vi "Testing.vi"() -> ()   [LabVIEW 2021]
uses:
  Motion_Panel_State_Machine/Motion_Panel_State_Machine.lvclass
  C:/Program Files (x86)/Hyper State Machine Framework/Hyper_Panel_State_Machine_Adaptive.lvlibp/Hyper Panel State Machine Object_Adaptive_2021/Hyper_Panel_State_Machine/Hyper_Panel_State_Machine_Adaptive.lvclass
  DIO_Panel_State_Machine/DIO_Panel_State_Machine.lvclass
  Class 1/Class 1.lvclass
  C:/Program Files (x86)/Hyper State Machine Framework/Hyper_Panel_State_Machine_Adaptive.lvlibp/Hyper Panel State Machine Object_Adaptive_2021/Panel_Core_Interface/Panel_Core_Interface.lvclass
  Class 2/Class 2.lvclass
  Class 3/Class 3.lvclass
  Project_Library/SSW_Hyper_State_Machine.lvlibp/State_Machine_Class/State_Machine_Module.llb/State Machine.ctl
  Project_Library/SSW_Hyper_State_Machine.lvlibp/State_Machine_Class/State_Machine_Module.llb/Lock_Unlock.ctl
  Project_Library/SSW_Hyper_State_Machine.lvlibp/State_Machine_Class/Main_State_Machine/Hyper_State_Machine.lvclass
  Project_Library/SSW_Hyper_State_Machine.lvlibp
panel:
  in  "Reset_All":bool
  in  "Change_VI_All":bool
  in  "Panel Index":i32=1 min=1 max=20
  in  "Implementation":u16(ring)
  in  "Change_VI":bool
  out "Main_Active":bool
  in  "Main_Interval(s)":dbl=0.05 format="%.0p"
  in  "Stop Button":bool=TRUE
  in  "Time Target (s)":dbl=30.0 format="%#_13g"
  in  "lock All":bool
  in  "Unlock":bool
  out "All_Values":variant[][](array[variant])
  out "error out":errorcluster
  in  "Exit":bool
  in  "Tab Control":T1(tab)
  out "Active 3":bool
  out "Active 2":bool
  out "Timing 3":dbl
  out "Timing 2":dbl
  out "Active 1":bool
  out "Timing 1":dbl
  out "Timing 4":dbl
  out "Active 4":bool
  # "Local"
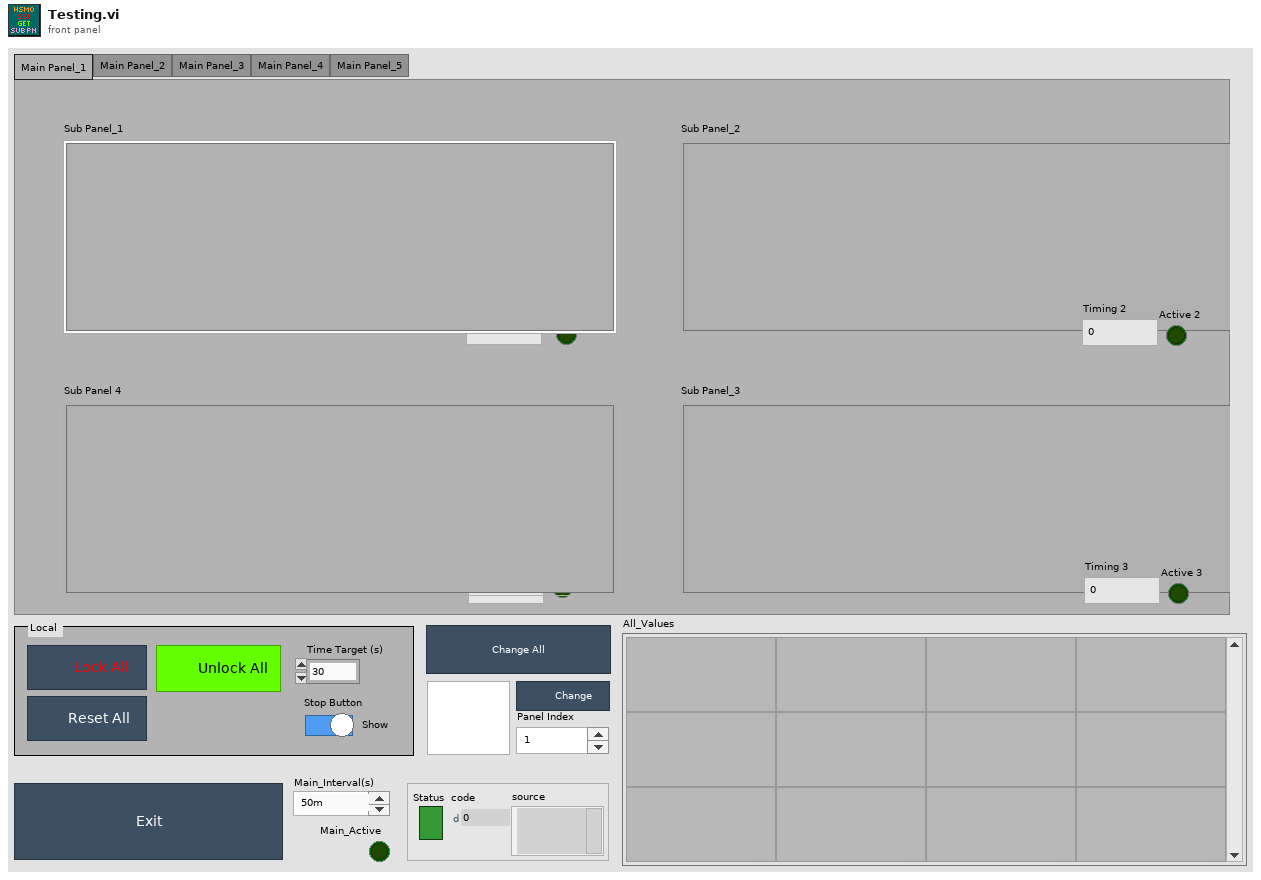
[diagram p1: front panel]
types:
  T1 = enum32{"Main Panel_1", "Main Panel_2", "Main Panel_3", "Main Panel_4", "Main Panel_5"}
  T2 = typedef "SSW_Hyper_State_Machine.lvlibp/State Machine.ctl" = cluster{"Command":string, "Data":variant}
  T3 = typedef "SSW_Hyper_State_Machine.lvlibp/Lock_Unlock.ctl" = cluster{"Action_Mode (Get)":enum16{"Set", "Get"}, "Action_Set (False)":bool, "State_In (Wait)":string}
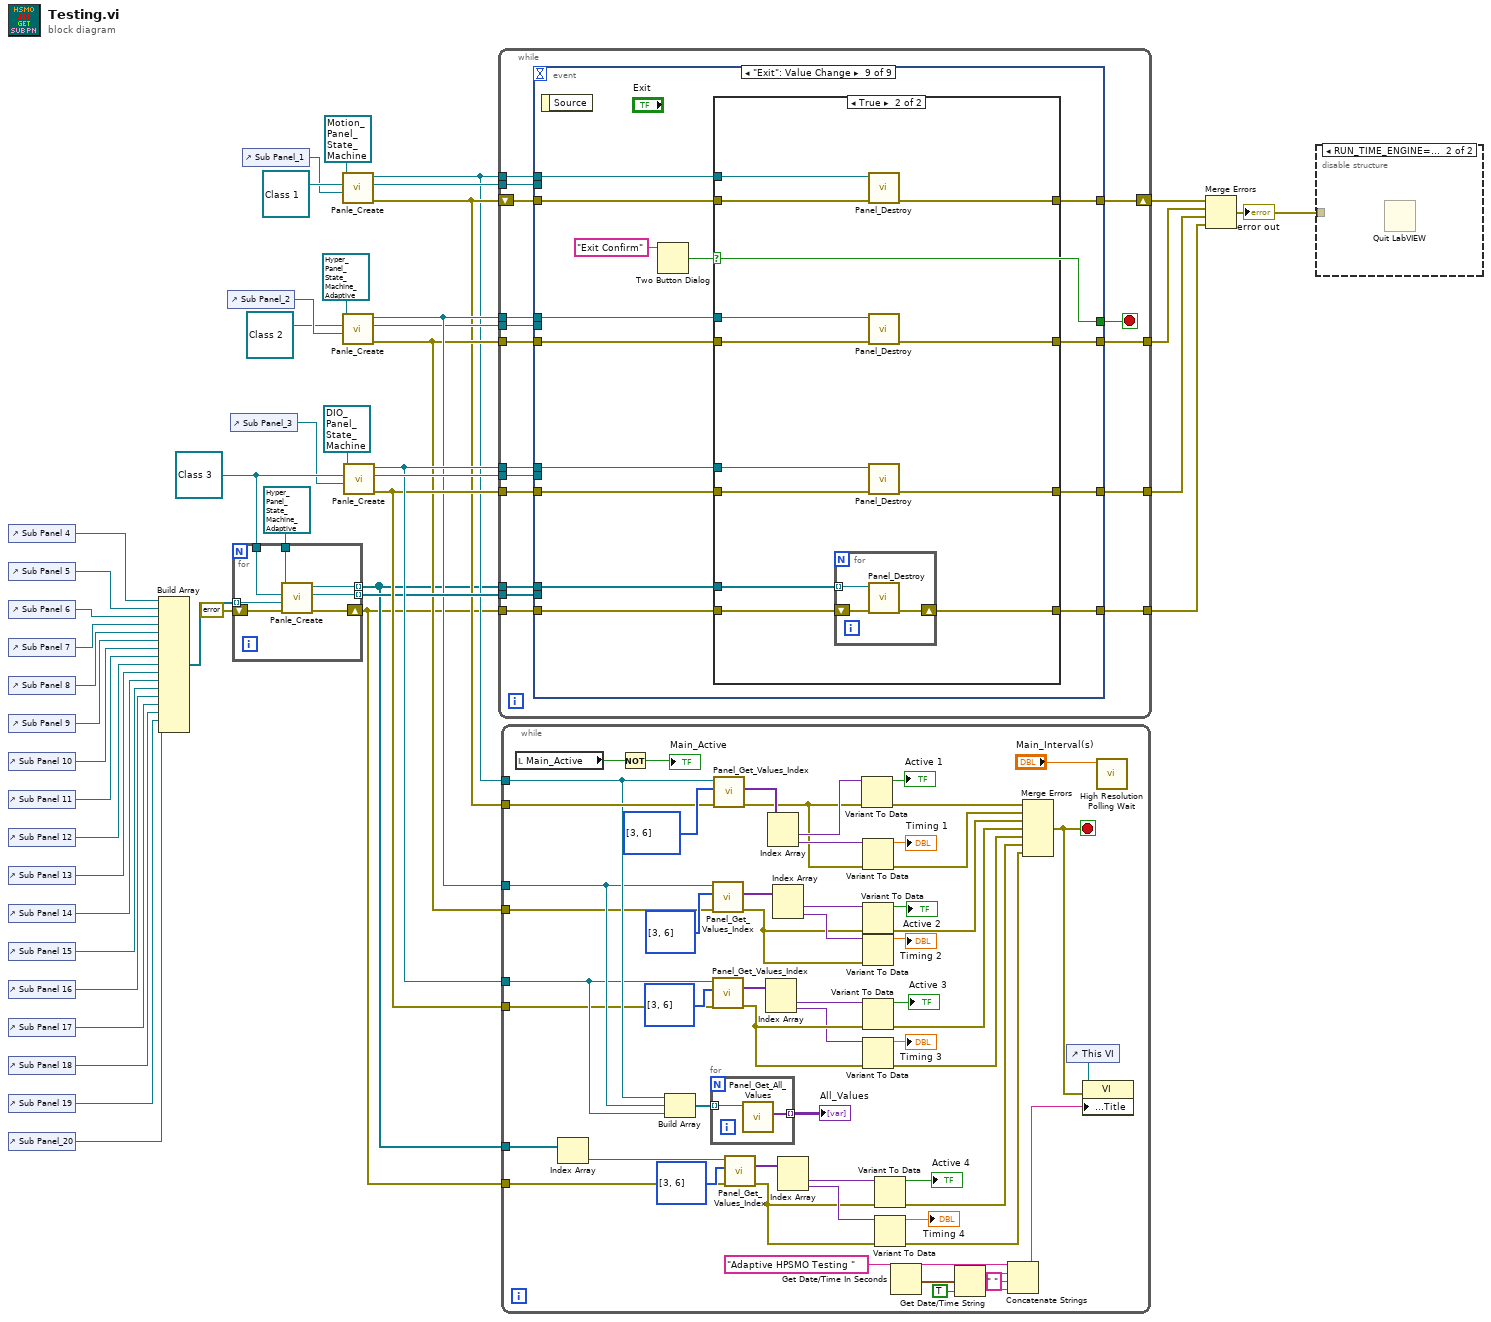
[diagram p0: block diagram]
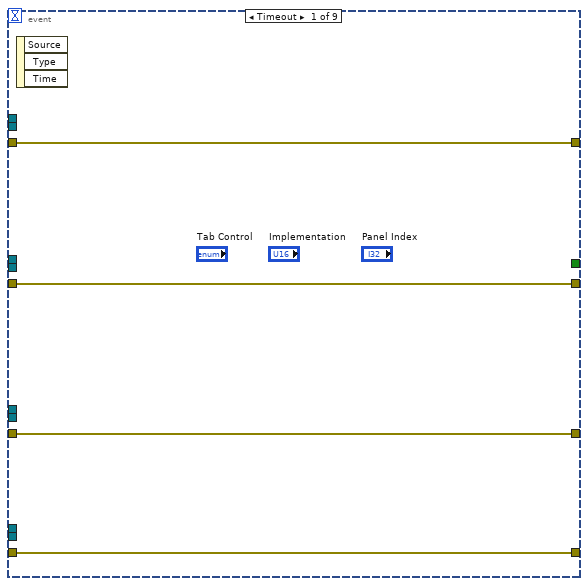
[diagram p3: hidden frame]
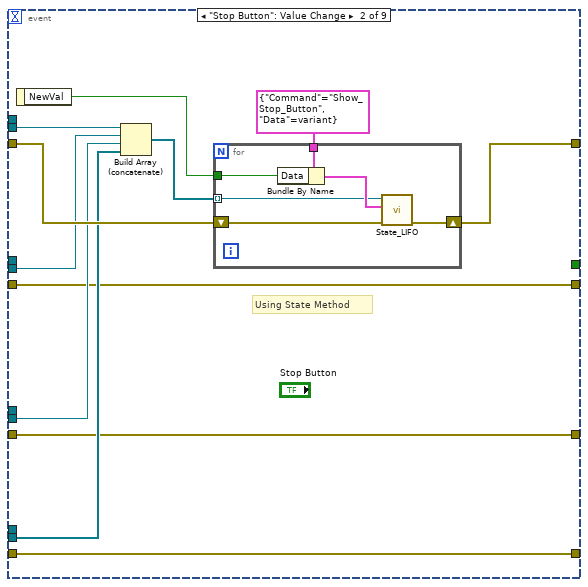
[diagram p4: hidden frame]
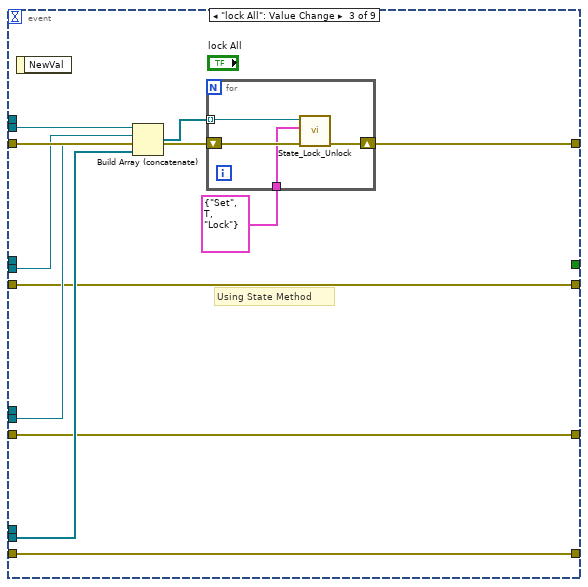
[diagram p5: hidden frame]
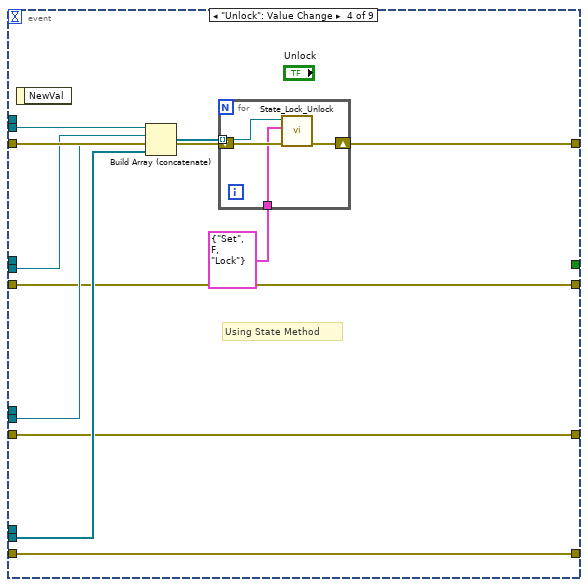
[diagram p6: hidden frame]
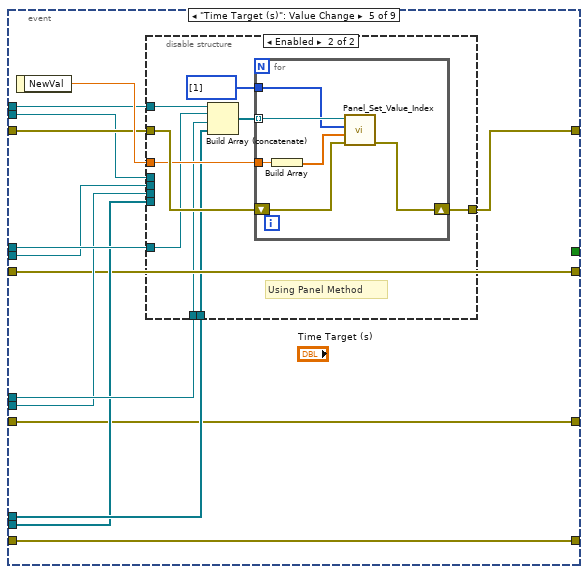
[diagram p7: hidden frame]
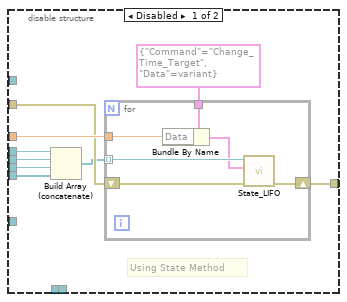
[diagram p8: hidden frame]
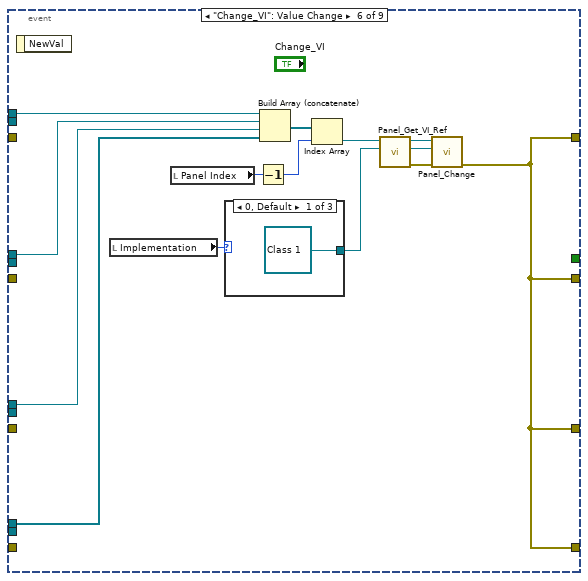
[diagram p9: hidden frame]
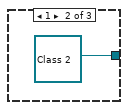
[diagram p10: hidden frame]
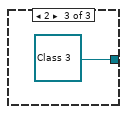
[diagram p11: hidden frame]
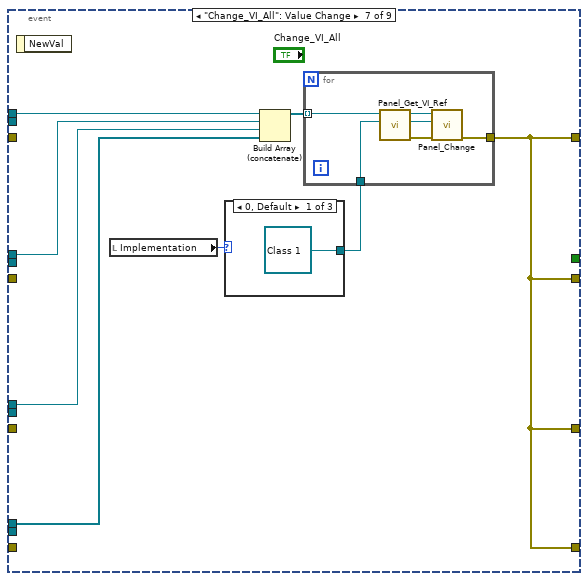
[diagram p12: hidden frame]
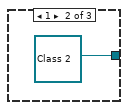
[diagram p13: hidden frame]
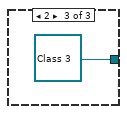
[diagram p14: hidden frame]
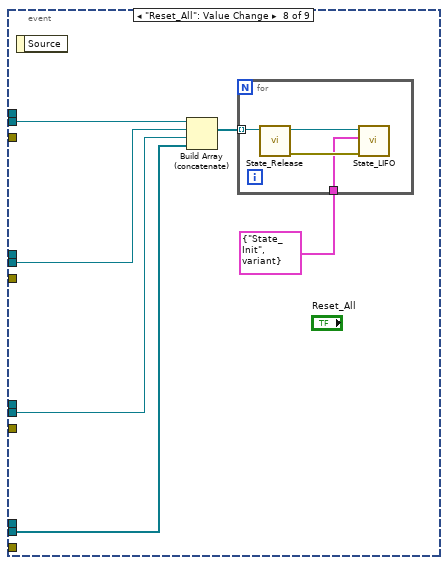
[diagram p15: hidden frame]
diagram:
  w7 = refnum<class "Class 3.lvclass"> refnum ("Class 3.lvclass")
  n1 = control-ref of="Sub Panel 4"() -> (w34:refnum<vi>)
  n2 = control-ref of="Sub Panel 5"() -> (w33:refnum<vi>)
  n3 = control-ref of="Sub Panel 6"() -> (w32:refnum<vi>)
  n4 = control-ref of="Sub Panel 7"() -> (w31:refnum<vi>)
  n5 = control-ref of="Sub Panel 8"() -> (w30:refnum<vi>)
  n6 = control-ref of="Sub Panel 9"() -> (w29:refnum<vi>)
  n7 = control-ref of="Sub Panel 10"() -> (w28:refnum<vi>)
  n8 = control-ref of="Sub Panel 11"() -> (w27:refnum<vi>)
  n9 = control-ref of="Sub Panel 12"() -> (w26:refnum<vi>)
  n10 = control-ref of="Sub Panel 13"() -> (w25:refnum<vi>)
  n11 = control-ref of="Sub Panel 14"() -> (w24:refnum<vi>)
  n12 = control-ref of="Sub Panel 15"() -> (w23:refnum<vi>)
  n13 = control-ref of="Sub Panel 16"() -> (w22:refnum<vi>)
  n14 = control-ref of="Sub Panel 17"() -> (w21:refnum<vi>)
  n15 = control-ref of="Sub Panel 18"() -> (w20:refnum<vi>)
  n16 = control-ref of="Sub Panel 19"() -> (w19:refnum<vi>)
  n17 = control-ref of="Sub Panel_20"() -> (w16:refnum<vi>)
  n18 = Build Array(w34, w33, w32, w31, w30, w29, w28, w27, w26, w25, w24, w23, w22, w21, w20, w19, w16) -> (w18:refnum<vi>[])
  n19 = control-ref of="Sub Panel_2"() -> (w8:refnum<vi>)
  n20 = control-ref of="Sub Panel_3"() -> (w6:refnum<vi>)
  n21 = for {
    tunnel: refnum<class "Hyper_Panel_State_Machine_Adaptive.lvclass"> refnum ("Hyper_Panel_State_Machine_Adaptive.lvlibp:Hyper_Panel_State_Machine_Adaptive.lvclass") -> [w53]
    tunnel: [w52] -> w2 mode=indexing
    shift-right: [w50] -> w1
    shift-left: errorcluster {"status"=FALSE, "code"=0, "source"=""} ("error out") -> [w51]
    tunnel: w18 -> [w48] mode=indexing
    tunnel: [w49] -> w17 mode=indexing
    tunnel: w7 -> [w47]
    n22 = call-dynamic "Panle_Create.vi"("error in (no error)"=w51, "Panel_Ref"=w48, "Panel_Core_Interface"=w47, "Hyper_Panel_State_Machine in"=w53) -> ("error out"=w50:errorcluster, "HSMO_Ref"=w49:refnum<class "Hyper_State_Machine.lvclass">, "Hyper_Panel_State_Machine out"=w52:refnum<class "Hyper_Panel_State_Machine_Adaptive.lvclass">)  [unwired: 5 in]
  }
  n23 = control-ref of="Sub Panel_1"() -> (w4:refnum<vi>)
  n24 = call-dynamic "Panle_Create.vi"("Panel_Ref"=w4, "Panel_Core_Interface"=refnum<class "Class 1.lvclass"> refnum ("Class 1.lvclass"), "Hyper_Panel_State_Machine in"=refnum<class "Motion_Panel_State_Machine.lvclass"> refnum ("Motion_Panel_State_Machine.lvclass")) -> ("error out"=w10:errorcluster, "HSMO_Ref"=w42:refnum<class "Hyper_State_Machine.lvclass">, "Hyper_Panel_State_Machine out"=w9:refnum<class "Motion_Panel_State_Machine.lvclass">)  [unwired: 6 in]
  n25 = call-dynamic "Panle_Create.vi"("Panel_Ref"=w8, "Panel_Core_Interface"=refnum<class "Class 2.lvclass"> refnum ("Class 2.lvclass"), "Hyper_Panel_State_Machine in"=refnum<class "Hyper_Panel_State_Machine_Adaptive.lvclass"> refnum ("Hyper_Panel_State_Machine_Adaptive.lvlibp:Hyper_Panel_State_Machine_Adaptive.lvclass")) -> ("error out"=w12:errorcluster, "HSMO_Ref"=w13:refnum<class "Hyper_State_Machine.lvclass">, "Hyper_Panel_State_Machine out"=w14:refnum<class "Hyper_Panel_State_Machine_Adaptive.lvclass">)  [unwired: 6 in]
  n26 = call-dynamic "Panle_Create.vi"("Panel_Ref"=w6, "Panel_Core_Interface"=w7, "Hyper_Panel_State_Machine in"=refnum<class "DIO_Panel_State_Machine.lvclass"> refnum ("DIO_Panel_State_Machine.lvclass")) -> ("error out"=w40:errorcluster, "HSMO_Ref"=w44:refnum<class "Hyper_State_Machine.lvclass">, "Hyper_Panel_State_Machine out"=w41:refnum<class "DIO_Panel_State_Machine.lvclass">)  [unwired: 6 in]
  n27 = while {
    shift-right: [w68] -> w46
    shift-left: w10 -> [w69]
    tunnel: w9 -> [w67]
    tunnel: w42 -> [w66]
    tunnel: [w60] -> w45
    tunnel: w12 -> [w61]
    tunnel: w13 -> [w65]
    tunnel: [w59] -> w43
    tunnel: w40 -> [w54]
    tunnel: w44 -> [w64]
    tunnel: w14 -> [w63]
    tunnel: w41 -> [w62]
    tunnel: w2 -> [w58]
    tunnel: w1 -> [w57]
    tunnel: [w56] -> w35
    tunnel: w17 -> [w55]
    stop <- w70 stop-if-true
    n28 = event shown="[8] \"Exit\": Value Change" {
      selector: _ -> [_ _ _ _ _ _ _ _ _]
      dyn-events: _ -> [_ _ _ _ _ _ _ _ _]
      timeout: _ -> [_ _ _ _ _ _ _ _ _]
      tunnel: [_ _ _ _ _ _ _ _ w223] -> w70
      tunnel: w69 -> [w74 w86 w102 w116 w133 _ _ _ w222]
      tunnel: [_ w85 w103 w118 w136 w170 w187 _ w217] -> w68
      tunnel: w67 -> [_ _ _ _ w134 w180 w191 _ w220]
      tunnel: w66 -> [_ w83 w101 w117 w132 _ _ w206 _]
      tunnel: w65 -> [_ w81 w99 w114 w129 _ _ w205 _]
      tunnel: w64 -> [_ w80 w98 w113 w128 _ _ w204 _]
      tunnel: w63 -> [_ _ _ _ w131 w179 w190 _ w221]
      tunnel: w62 -> [_ _ _ _ w130 w178 w189 _ w219]
      tunnel: w61 -> [w71 w77 w95 w110 w123 _ _ _ w214]
      tunnel: [w74 _ _ _ _ _ _ _ _] -> _
      tunnel: [w71 w77 w95 w110 w123 w170 w187 _ w216] -> w60
      tunnel: [w72 w76 w94 w109 w124 w170 w187 _ w215] -> w59
      tunnel: w58 -> [_ _ _ _ w127 w177 w188 _ w213]
      tunnel: w57 -> [w73 w75 w93 w108 w125 _ _ _ w212]
      tunnel: [w73 w75 w93 w108 w125 w170 w187 _ w211] -> w56
      tunnel: w55 -> [_ w78 w96 w111 w126 _ _ w203 _]
      tunnel: w54 -> [w72 w76 w94 w109 w124 _ _ _ w218]
      event Timeout {
        n29 = event-data() -> ()  [unwired: 1 in, 3 out]
      }
      event "Stop Button": Value Change {
        # "Using State Method"
        n30 = event-data() -> ("NewVal"=w84:bool)  [unwired: 1 in]
        n31 = Build Array (concatenate)(w83, w81, w80, w78) -> (w82:refnum<class "Hyper_State_Machine.lvclass">[])
        n32 = for {
          tunnel: w84 -> [w90]
          tunnel: w82 -> [w88] mode=indexing
          shift-right: [w91] -> w85
          shift-left: w86 -> [w92]
          tunnel: T2 {"Command"="Show_Stop_Button", "Data"=variant} ("State Machine") -> [w87]
          n33 = Bundle By Name(cluster=w87, "Data"=w90) -> (w89:T2)
          n34 = call-dynamic "State_LIFO.vi"("error in (no error)"=w92, "State Machine"=w89, "State_Machine_Class in"=w88) -> ("error out"=w91:errorcluster)  [unwired: 7 in, 1 out]
        }
      }
      event "lock All": Value Change {
        # "Using State Method"
        n35 = event-data() -> ()  [unwired: 1 in, 1 out]
        n36 = Build Array (concatenate)(w101, w99, w98, w96) -> (w100:refnum<class "Hyper_State_Machine.lvclass">[])
        n37 = for {
          tunnel: w100 -> [w105] mode=indexing
          shift-right: [w107] -> w103
          shift-left: w102 -> [w106]
          tunnel: T3 {"Action_Mode (Get)"=enum."Set", "Action_Set (False)"=TRUE, "State_In (Wait)"="Lock"} ("Parameter") -> [w104]
          n38 = call-dynamic "State_Lock_Unlock.vi"("error in (no error)"=w106, "Parameter"=w104, "State_Machine_Class in"=w105) -> ("error out"=w107:errorcluster)  [unwired: 6 in, 2 out]
        }
      }
      event "Unlock": Value Change {
        # "Using State Method"
        n39 = event-data() -> ()  [unwired: 1 in, 1 out]
        n40 = Build Array (concatenate)(w117, w114, w113, w111) -> (w115:refnum<class "Hyper_State_Machine.lvclass">[])
        n41 = for {
          tunnel: w115 -> [w121] mode=indexing
          shift-right: [w122] -> w118
          shift-left: w116 -> [w120]
          tunnel: T3 {"Action_Mode (Get)"=enum."Set", "Action_Set (False)"=FALSE, "State_In (Wait)"="Lock"} ("Parameter") -> [w119]
          n42 = call-dynamic "State_Lock_Unlock.vi"("error in (no error)"=w120, "Parameter"=w119, "State_Machine_Class in"=w121) -> ("error out"=w122:errorcluster)  [unwired: 6 in, 2 out]
        }
      }
      event "Time Target (s)": Value Change {
        n43 = event-data() -> ("NewVal"=w135:dbl)  [unwired: 1 in]
        n44 = disable-structure shown="Enabled" {
          disable-tunnel: w132 -> [w144 _]
          disable-tunnel: [w143 w157] -> w136
          disable-tunnel: w135 -> [w145 w158]
          disable-tunnel: w134 -> [_ w160]
          disable-tunnel: w133 -> [w142 w159]
          disable-tunnel: w131 -> [_ w155]
          disable-tunnel: w130 -> [_ w154]
          disable-tunnel: w129 -> [w140 _]
          disable-tunnel: w128 -> [w139 _]
          disable-tunnel: w127 -> [_ w152]
          disable-tunnel: w126 -> [w137 _]
          frame Disabled {
            # "Using State Method"
            n45 = Build Array (concatenate)(w144, w140, w139, w137) -> (w141:refnum<class "Hyper_State_Machine.lvclass">[])
            n46 = for {
              tunnel: w145 -> [w151]
              tunnel: w141 -> [w150] mode=indexing
              shift-right: [w149] -> w143
              shift-left: w142 -> [w147]
              tunnel: T2 {"Command"="Change_Time_Target", "Data"=variant} ("State Machine") -> [w146]
              n47 = Bundle By Name(cluster=w146, "Data"=w151) -> (w148:T2)
              n48 = call-dynamic "State_LIFO.vi"("error in (no error)"=w147, "State Machine"=w148, "State_Machine_Class in"=w150) -> ("error out"=w149:errorcluster)  [unwired: 7 in, 1 out]
            }
          }
          frame Enabled {
            # "Using Panel Method"
            n49 = Build Array (concatenate)(w160, w155, w154, w152) -> (w156:refnum<class "Hyper_Panel_State_Machine_Adaptive.lvclass">[])
            n50 = for {
              tunnel: w156 -> [w165] mode=indexing
              tunnel: w158 -> [w166]
              shift-right: [w161] -> w157
              shift-left: w159 -> [w162]
              tunnel: i32[] [1] ("Control_Indexes(Tabbing Order)") -> [w164]
              n51 = Build Array(w166) -> (w163:dbl[])
              n52 = call-dynamic "Panel_Set_Value_Index.vi"("error in (no error)"=w162, "Data_Values"=w163, "Control_Indexes(Tabbing Order)"=w164, "Hyper_Panel_State_Machine in"=w165) -> ("error out"=w161:errorcluster)  [unwired: 6 in, 1 out]
            }
          }
        }
      }
      event "Change_VI": Value Change {
        n53 = event-data() -> ()  [unwired: 1 in, 1 out]
        n54 = local read "Implementation"() -> (w167:u16)
        n55 = local read "Panel Index"() -> (w168:i32)
        n56 = case shown="0, Default" w167 {
          tunnel: [refnum<class "Class 1.lvclass"> refnum ("Class 1.lvclass") refnum<class "Class 2.lvclass"> refnum ("Class 2.lvclass") refnum<class "Class 3.lvclass"> refnum ("Class 3.lvclass")] -> w169
          frame 0, Default {
          }
          frame 1 {
          }
          frame 2 {
          }
        }
        n57 = Decrement(x=w168) -> (x-1=w175:i32)
        n58 = Build Array (concatenate)(w180, w179, w178, w177) -> (w176:refnum<class "Hyper_Panel_State_Machine_Adaptive.lvclass">[])
        n59 = Index Array(array=w176, index=w175) -> (element=w174:refnum<class "Hyper_Panel_State_Machine_Adaptive.lvclass">)
        n60 = call-dynamic "Panel_Get_VI_Ref.vi"("Panel_Core_Interface"=w169, "Hyper_Panel_State_Machine_Adaptive in"=w174) -> ("error out"=w171:errorcluster, "Core_VI_Ref"=w172:refnum<vi>, "Hyper_Panel_State_Machine_Adaptive out"=w173:refnum<class "Hyper_Panel_State_Machine_Adaptive.lvclass">)  [unwired: 7 in]
        n61 = call-dynamic "Panel_Change.vi"("error in (no error)"=w171, "Core_VI_Ref"=w172, "Hyper_Panel_State_Machine in"=w173) -> ("error out"=w170:errorcluster)  [unwired: 7 in, 1 out]
      }
      event "Change_VI_All": Value Change {
        n62 = event-data() -> ()  [unwired: 1 in, 1 out]
        n63 = local read "Implementation"() -> (w185:u16)
        n64 = case shown="0, Default" w185 {
          tunnel: [refnum<class "Class 1.lvclass"> refnum ("Class 1.lvclass") refnum<class "Class 2.lvclass"> refnum ("Class 2.lvclass") refnum<class "Class 3.lvclass"> refnum ("Class 3.lvclass")] -> w186
          frame 0, Default {
          }
          frame 1 {
          }
          frame 2 {
          }
        }
        n65 = Build Array (concatenate)(w191, w190, w189, w188) -> (w184:refnum<class "Hyper_Panel_State_Machine_Adaptive.lvclass">[])
        n66 = for {
          tunnel: [w194] -> w187
          tunnel: w186 -> [w193]
          tunnel: w184 -> [w192] mode=indexing
          n67 = call-dynamic "Panel_Get_VI_Ref.vi"("Panel_Core_Interface"=w193, "Hyper_Panel_State_Machine_Adaptive in"=w192) -> ("error out"=w195:errorcluster, "Core_VI_Ref"=w196:refnum<vi>, "Hyper_Panel_State_Machine_Adaptive out"=w197:refnum<class "Hyper_Panel_State_Machine_Adaptive.lvclass">)  [unwired: 7 in]
          n68 = call-dynamic "Panel_Change.vi"("error in (no error)"=w195, "Core_VI_Ref"=w196, "Hyper_Panel_State_Machine in"=w197) -> ("error out"=w194:errorcluster)  [unwired: 7 in, 1 out]
        }
      }
      event "Reset_All": Value Change {
        n69 = event-data() -> ()  [unwired: 1 in, 1 out]
        n70 = Build Array (concatenate)(w206, w205, w204, w203) -> (w202:refnum<class "Hyper_State_Machine.lvclass">[])
        n71 = for {
          tunnel: w202 -> [w210] mode=indexing
          tunnel: T2 {"Command"="State_Init", "Data"=variant} ("State Machine") -> [w207]
          n72 = call-dynamic "State_Release.vi"("State_Machine_Class in"=w210) -> ("error out"=w208:errorcluster, "State_Machine_Class out"=w209:refnum<class "Hyper_State_Machine.lvclass">)  [unwired: 9 in]
          n73 = call-dynamic "State_LIFO.vi"("error in (no error)"=w208, "State Machine"=w207, "State_Machine_Class in"=w209) -> ()  [unwired: 7 in, 2 out]
        }
      }
      event "Exit": Value Change {
        n74 = event-data() -> ()  [unwired: 1 in, 1 out]
        n75 = Two Button Dialog(message="Exit Confirm") -> (T button?=w223:bool)  [unwired: 2 in]
        n76 = case shown="True" w223 {
          tunnel: w222 -> [w228 w240]
          tunnel: w221 -> [_ w231]
          tunnel: w220 -> [_ w239]
          tunnel: w219 -> [_ w238]
          tunnel: w218 -> [w226 w237]
          tunnel: [w228 w236] -> w217
          tunnel: [w227 w229] -> w216
          tunnel: [w226 w235] -> w215
          tunnel: w214 -> [w227 w230]
          tunnel: w213 -> [_ w234]
          tunnel: w212 -> [w225 w233]
          tunnel: [w225 w232] -> w211
          frame False {
          }
          frame True {
            n77 = for {
              tunnel: w234 -> [w243] mode=indexing
              shift-right: [w241] -> w232
              shift-left: w233 -> [w242]
              n78 = call-dynamic "Panel_Destroy.vi"("error in (no error)"=w242, "Hyper_Panel_State_Machine in"=w243) -> ("error out"=w241:errorcluster)  [unwired: 9 in]
            }
            n79 = call-dynamic "Panel_Destroy.vi"("error in (no error)"=w240, "Hyper_Panel_State_Machine in"=w239) -> ("error out"=w236:errorcluster)  [unwired: 9 in]
            n80 = call-dynamic "Panel_Destroy.vi"("error in (no error)"=w230, "Hyper_Panel_State_Machine in"=w231) -> ("error out"=w229:errorcluster)  [unwired: 9 in]
            n81 = call-dynamic "Panel_Destroy.vi"("error in (no error)"=w237, "Hyper_Panel_State_Machine in"=w238) -> ("error out"=w235:errorcluster)  [unwired: 9 in]
          }
        }
      }
    }
  }
  n82 = while {
    tunnel: w9 -> [w273]
    tunnel: w14 -> [w262]
    tunnel: w41 -> [w257]
    tunnel: w10 -> [w279]
    tunnel: w12 -> [w260]
    tunnel: w40 -> [w256]
    tunnel: w2 -> [w250]
    tunnel: w1 -> [w246]
    stop <- w264 stop-if-true
    n83 = local read "Main_Active"() -> (w277:bool)
    n84 = Index Array(array=w250) -> (element=w249:refnum<class "Hyper_Panel_State_Machine_Adaptive.lvclass">)  [unwired: 1 in]
    n85 = Not(x=w277) -> (.not. x?=→"Main_Active":bool)
    n86 = Build Array(w273, w262, w257) -> (w274:refnum<class "Hyper_Panel_State_Machine_Adaptive.lvclass">[])
    n87 = for {
      tunnel: w274 -> [w303] mode=indexing
      tunnel: [w302] -> w272 mode=indexing
      n88 = call-dynamic "Panel_Get_All_Values.vi"("Hyper_Panel_State_Machine in"=w303) -> ("All_Values"=w302:variant[])  [unwired: 8 in, 2 out]
    }
    "All_Values" <- w272
    n89 = call-dynamic "Panel_Get_Values_Index.vi"("error in (no error)"=w260, "Control_Indexes(Tabbing Order)"=i32[] [3, 6], "Hyper_Panel_State_Machine in"=w262) -> ("error out"=w258:errorcluster, "Data_Values"=w259:variant[])  [unwired: 6 in, 1 out]
    n90 = call-dynamic "Panel_Get_Values_Index.vi"("error in (no error)"=w256, "Control_Indexes(Tabbing Order)"=i32[] [3, 6], "DIO_Panel_State_Machine in"=w257) -> ("error out"=w301:errorcluster, "Data_Values"=w289:variant[])  [unwired: 6 in, 1 out]
    n91 = call-dynamic "Panel_Get_Values_Index.vi"("error in (no error)"=w279, "Control_Indexes(Tabbing Order)"=i32[] [3, 6] ("control indexes"), "Motion_Panel_State_Machine in"=w273) -> ("error out"=w275:errorcluster, "Data_Values"=w288:variant[])  [unwired: 6 in, 1 out]
    n92 = call-dynamic "Panel_Get_Values_Index.vi"("error in (no error)"=w246, "Control_Indexes(Tabbing Order)"=i32[] [3, 6], "Hyper_Panel_State_Machine in"=w249) -> ("error out"=w251:errorcluster, "Data_Values"=w254:variant[])  [unwired: 6 in, 1 out]
    n93 = Index Array(array=w289) -> (element #1=w295:variant, element #2=w293:variant)  [unwired: 2 in]
    n94 = Index Array(array=w288) -> (element #1=w282:variant, element #2=w284:variant)  [unwired: 2 in]
    n95 = Index Array(array=w259) -> (element #1=w294:variant, element #2=w292:variant)  [unwired: 2 in]
    n96 = Index Array(array=w254) -> (element #1=w252:variant, element #2=w253:variant)  [unwired: 2 in]
    n97 = Variant To Data(error in=w275, Variant=w282) -> (data=→"Active 1":bool, error out=w286:errorcluster)  [unwired: 1 in]
    n98 = Variant To Data(error in=w275, Variant=w284) -> (data=→"Timing 1":dbl, error out=w287:errorcluster)  [unwired: 1 in]
    n99 = Variant To Data(error in=w258, Variant=w294) -> (data=→"Active 2":bool, error out=w298:errorcluster)  [unwired: 1 in]
    n100 = Variant To Data(error in=w258, Variant=w292) -> (data=→"Timing 2":dbl)  [unwired: 1 in, 1 out]
    n101 = Variant To Data(error in=w301, Variant=w295) -> (data=→"Active 3":bool, error out=w299:errorcluster)  [unwired: 1 in]
    n102 = Variant To Data(error in=w301, Variant=w293) -> (data=→"Timing 3":dbl, error out=w300:errorcluster)  [unwired: 1 in]
    n103 = Variant To Data(error in=w251, Variant=w252) -> (data=→"Active 4":bool, error out=w245:errorcluster)  [unwired: 1 in]
    n104 = Variant To Data(error in=w251, Variant=w253) -> (data=→"Timing 4":dbl, error out=w244:errorcluster)  [unwired: 1 in]
    n105 = Get Date/Time In Seconds() -> (seconds since 1Jan1904=w271:timestamp)
    n106 = Get Date/Time String(seconds (now)=w271, want seconds? (F)=TRUE) -> (date string=w269:string, time string=w265:string)  [unwired: 1 in]
    n107 = Concatenate Strings("Adaptive HPSMO Testing " ("string"), w269, " " ("string"), w265) -> (w267:string)
    n108 = Merge Errors(w286, w287, w298, w299, w300, w245, w244) -> (w264:errorcluster)
    n109 = control-ref of="This VI"() -> (w263:refnum<vi>)
    n110 = property class="VI"(reference=w263, error in=w264, "Front Panel.Title"=w267) -> ()  [unwired: 2 out]
    n111 = call <vilib>:"High Resolution Polling Wait.vi"("seconds to wait"="Main_Interval(s)") -> ()  [unwired: 10 in, 1 out]
  }
  n112 = Merge Errors(w46, w45, w43, w35) -> (w37:errorcluster)
  "error out" <- w37
  n113 = disable-structure shown="RUN_TIME_ENGINE==True" {
    disable-tunnel: w37 -> [_ _]
    frame condition #0 (active) {
    }
    frame condition #1 {
      n114 = Quit LabVIEW() -> ()  [unwired: 1 in]
    }
  }
